vi "Take single measurement.vi"() -> ()   [LabVIEW 2017, in "GP22_TDC_Arduinoed.lvlib"]
uses:
  GP22_TDC_Arduinoed.lvlib
panel:
  out "error out":errorcluster
  out "Calibration / s":dbl format="%^#_6g"
  out "output / s":dbl format="%^#_6g"
  out "Freq / Hz":dbl
  out "Self-Test Result Message":string
  in  "VISA resource name":refnum<visa-resource-name>
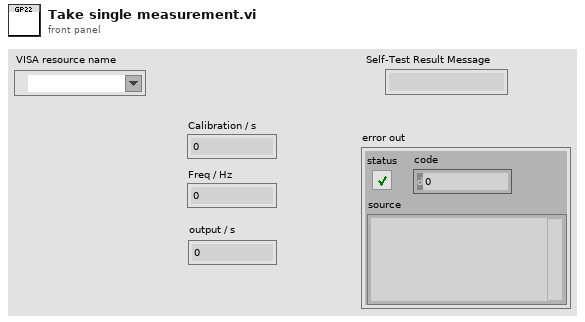
[diagram p1: front panel]
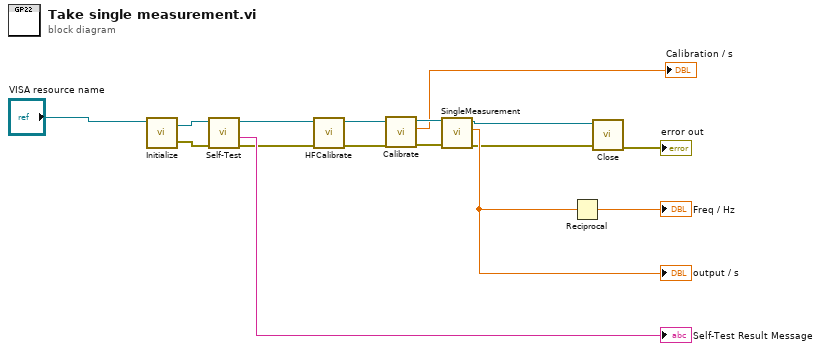
[diagram p0: block diagram]
diagram:
  n1 = call "Initialize.vi"("VISA resource name"="VISA resource name") -> ("error out"=w14:errorcluster, "VISA resource name out"=w15:refnum<visa-resource-name>)  [unwired: 5 in]
  n2 = call "Self-Test.vi"("error in (no error)"=w14, "VISA resource name"=w15) -> ("error out"=w3:errorcluster, "Self-Test Result Message"=→"Self-Test Result Message":string, "VISA resource name out"=w2:refnum<visa-resource-name>)  [unwired: 6 in, 1 out]
  n3 = call "HFCalibrate.vi"("error in (no error)"=w3, "VISA resource name"=w2) -> ("error out"=w4:errorcluster, "VISA resource name out"=w5:refnum<visa-resource-name>)  [unwired: 5 in, 2 out]
  n4 = call "Calibrate.vi"("error in (no error)"=w4, "VISA resource name"=w5) -> ("error out"=w8:errorcluster, "output / s"=→"Calibration / s":dbl, "VISA resource name out"=w9:refnum<visa-resource-name>)  [unwired: 5 in, 1 out]
  n5 = call "SingleMeasurement.vi"("error in (no error)"=w8, "VISA resource name"=w9) -> ("error out"=w7:errorcluster, "output / s"=w10:dbl, "VISA resource name out"=w12:refnum<visa-resource-name>)  [unwired: 7 in]
  "output / s" <- w10
  n6 = Reciprocal(x=w10) -> (1/x=→"Freq / Hz":dbl)
  n7 = call "Close.vi"("error in (no error)"=w7, "VISA resource name"=w12) -> ("error out"=→"error out":errorcluster)  [unwired: 9 in]
